vi "SSL_CTX_set_verify.vi"(8 "error in (no error)":errorcluster, 10 "Mode":T1 items=["SSL_VERIFY_NONE"=0, "SSL_VERIFY_PEER"=1, "SSL_VERIFY_FAIL_IF_NO_PEER_CERT"=2, "SSL_VERIFY_CLIENT_ONCE"=4], 11 "SSL-Context in":refnum<class "SSL-Context.lvclass">) -> (0 "error out":errorcluster, 3 "SSL-Context out":refnum<class "SSL-Context.lvclass">)   [LabVIEW 2013, in "SSL_Lib.lvlib" / "SSL-Context.lvclass"]
uses:
  SSL-Context.lvclass
  SSL Verify Mode.ctl
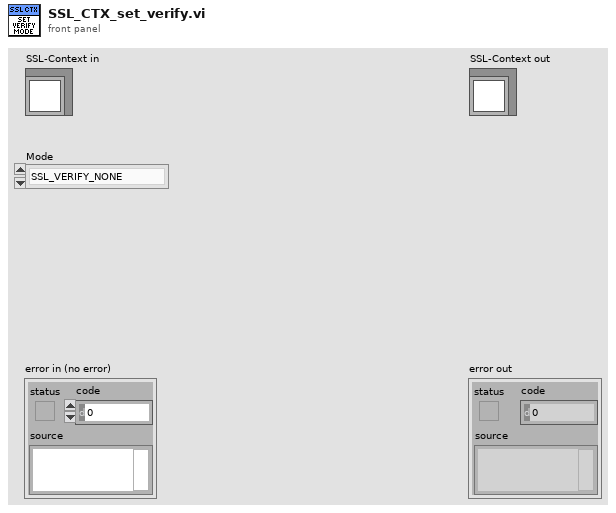
[diagram p1: front panel]
types:
  T1 = typedef "SSL_Lib.lvlib/SSL-Context.lvclass/SSL Verify Mode.ctl" = i32
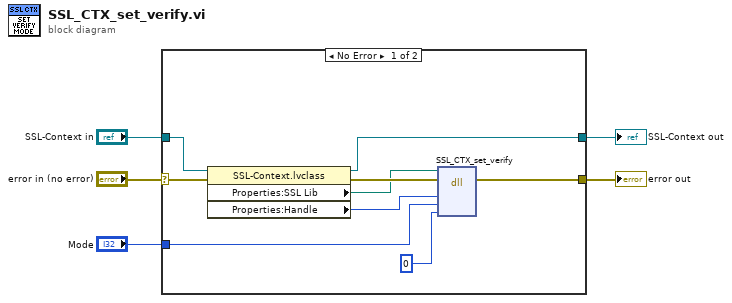
[diagram p0: block diagram]
diagram:
  n1 = case shown="No Error" "error in (no error)" {
    selector: "error in (no error)" -> [w14 w16]
    tunnel: [w9 w16] -> w4
    tunnel: [w8 w15] -> w2
    tunnel: "SSL-Context in" -> [w12 w15]
    tunnel: "Mode" -> [w6 _]
    frame No Error {
      n2 = property class="SSL-Context.lvclass"(reference=w12, error in=w14) -> (reference out=w8:refnum<class "SSL-Context.lvclass">, error out=w13:errorcluster, "Properties:SSL Lib"=w11:path, "Properties:Handle"=w10:u64)
      n3 = dll-call lib="C:/Program Files (x86)/National Instruments/Shared/nissl/NIssleay32.dll" fn="SSL_CTX_set_verify"(path in=w11, error in=w13, "SSL_CTX"=w10, "mode"=w6, "callback"=0 ("arg2")) -> (error out=w9:errorcluster)  [unwired: 5 in, 1 out]
    }
    frame Error {
    }
  }
  "error out" <- w4
  "SSL-Context out" <- w2
